vi "FTW-JSON-LexicalScan-Space.vi"(0 "JSON String":string, 7 "JSON Parent":T1, 9 "Starting Offset":i32, 11 "error in":errorcluster) -> (4 "JSON String Out":string, 6 "JSON Part":T1, 8 "Container":variant, 10 "Offset after Match":i32, 14 "Found Match?":bool, 15 "error out":errorcluster)   [LabVIEW 2015]
uses:
  FTW-JSON-Part.ctl
panel:
  # "Inputs"
  # "Outputs"
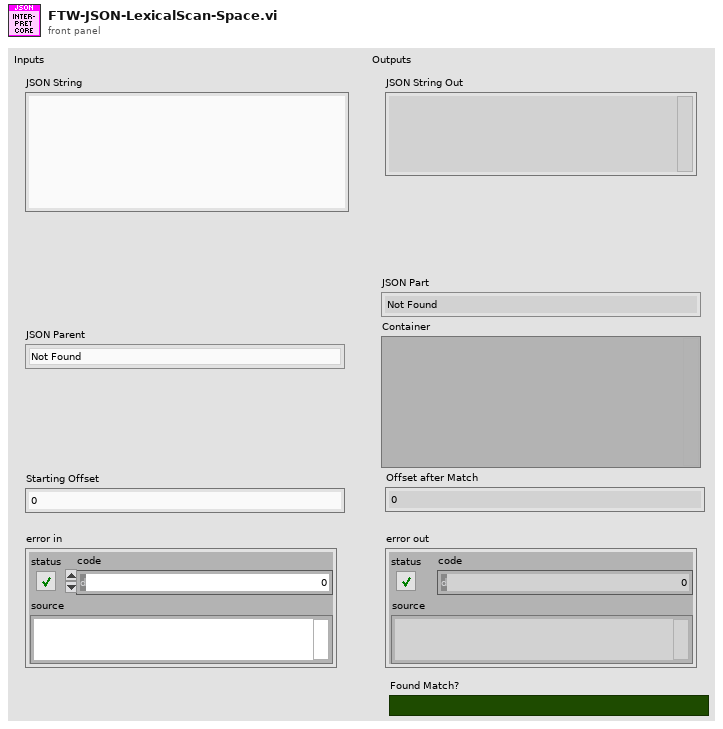
[diagram p1: front panel]
types:
  T1 = typedef "FTW-JSON-Part.ctl" = enum8{"Not Found", "Object", "Object Inner", "Array", "Array Inner", "String", "Number", "Boolean", "null"}
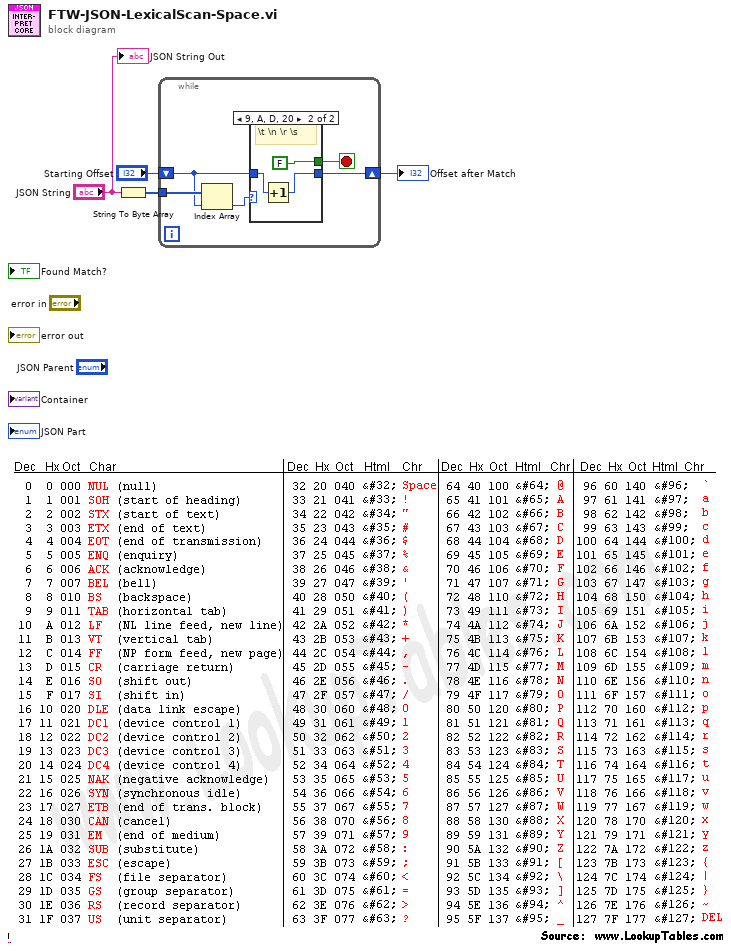
[diagram p0: block diagram]
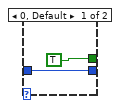
[diagram p2: hidden frame]
diagram:
  n1 = String To Byte Array(string="JSON String") -> (unsigned byte array=w3:u8[])
  n2 = while {
    shift-right: [w6] -> w2
    shift-left: "Starting Offset" -> [w5]
    tunnel: w3 -> [w9]
    stop <- w7 stop-if-true
    n3 = Index Array(array=w9, index=w5) -> (element=w8:u8)
    n4 = case shown="9, A, D, 20" w8 {
      tunnel: [TRUE FALSE] -> w7
      tunnel: [w10 w13] -> w6
      tunnel: w5 -> [w10 w12]
      frame 0, Default {
      }
      frame 9, 10, 13, 32 {
        # "\\t \\n \\r \\s"
        n5 = Increment(x=w12) -> (x+1=w13:i32)
      }
    }
  }
  "Offset after Match" <- w2
  "JSON String Out" <- "JSON String"
